vi "max (SubVI).vi"(10 "initialized array":fxp<+/-,64,32>[](array[numeric])) -> (2 "y":fxp<+/-,64,32>)   [LabVIEW 2017]
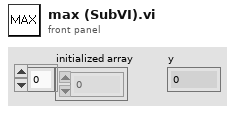
[diagram p1: front panel]
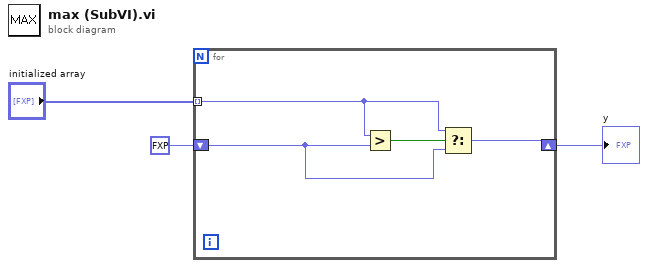
[diagram p0: block diagram]
diagram:
  n1 = for {
    tunnel: "initialized array" -> [w6] mode=indexing
    shift-right: [w4] -> w1
    shift-left: fxp<+,1,1> 0.0 ("y") -> [w5]
    n2 = Greater?(x=w6, y=w5) -> (0:w7:bool)
    n3 = Select(t=w6, s=w7, f=w5) -> (s? t:f=w4:fxp<+/-,64,32>)
  }
  "y" <- w1
